vi "thruster_enable_set.vi"(8 "enable":bool, 9 "index":u16, 10 "Address":u16, 11 "VISA resource name":refnum<visa-resource-name>) -> ()   [LabVIEW 2014]
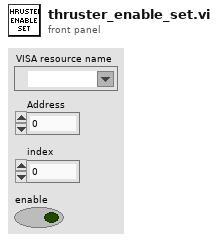
[diagram p1: front panel]
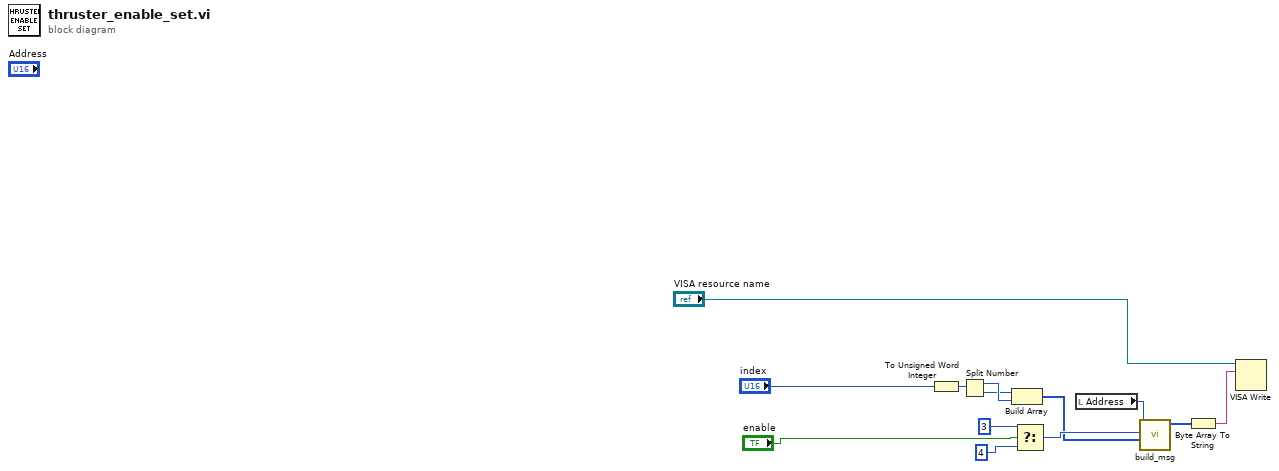
[diagram p0: block diagram]
diagram:
  n1 = To Unsigned Word Integer(number="index") -> (unsigned 16bit integer=w9:u16)
  n2 = Split Number(x=w9) -> (hi(x)=w7:u8, lo(x)=w6:u8)
  n3 = Build Array(w6, w7) -> (w8:u8[])
  n4 = Select(t=u16 3 ("ID"), s="enable", f=u16 4 ("ID")) -> (s? t:f=w12:u16)
  n5 = local read "Address"() -> (w13:u16)
  n6 = call "build_msg.vi"("data"=w8, "ID"=w12, "Address"=w13) -> ("msg"=w5:u8[])  [unwired: 8 in]
  n7 = Byte Array To String(unsigned byte array=w5) -> (string=w4:string)
  n8 = VISA Write(VISA resource name="VISA resource name", write buffer=w4) -> ()  [unwired: 1 in, 3 out]
